vi "Autonomous_Execution.vi"(0 "Queue Key":refnum<queue>, 5 "Autonomous_Queue":refnum<queue>, 11 "error in":errorcluster) -> (6 "Done":bool)   [LabVIEW 2019]
uses:
  Queue_Key_Data.ctl
  Robot_Subsystems.ctl
  Subsystems/Drive/Drive_Cluster.ctl
  Subsystems/Drive/Drive_Control_States.ctl
  Subsystems/Drive/Drive_Orientation_States.ctl
  Subsystems/Intake/Intake_Cluster.ctl
  Subsystems/Intake/Intake_States.ctl
  Globals/Drive_Globals.vi
  Globals/Intake_Globals.vi
panel:
  in  "ignore previous (F)":bool
  in  "timeout in ms (-1)":i32=15
  out "notifiers out":refnum<notifier>[](array[refnum])
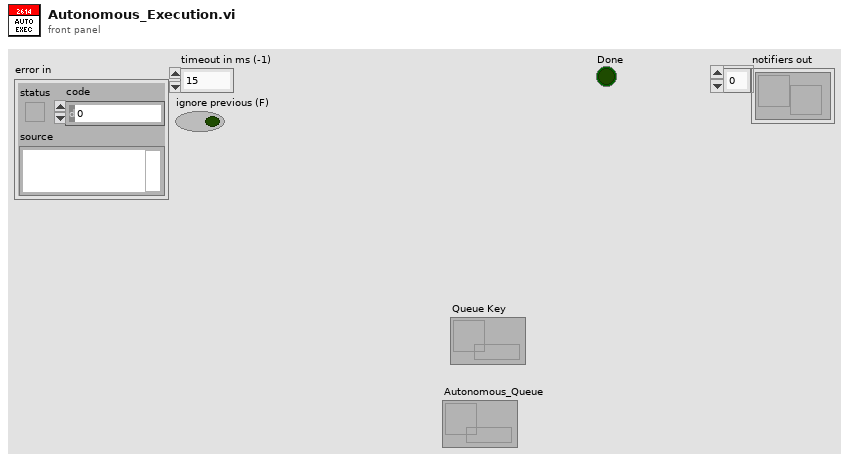
[diagram p1: front panel]
types:
  T1 = typedef "Queue_Key_Data.ctl" = cluster{"Operation Notifier":refnum<notifier>, "Subsystem":string, "Concurrent":bool}
  T2 = typedef "Robot_Subsystems.ctl" = cluster{"Drive_Cluster":T3, "Intake_Cluster":T6}
  T3 = typedef "Drive_Cluster.ctl" = cluster{"Control_State":T4, "Vertical_Throttle":dbl, "Lateral_Throttle":dbl, "Rotational_Throttle":dbl, "Strafe_In_Deadband":bool, "Rotation_In_Deadband":bool, "Orientation_State":T5, "Parameters":dbl[], "Step":i32, "Auto_Notifier":refnum<notifier>, "PathName":string}
  T4 = typedef "Drive_Control_States.ctl" = enum16{"No-Op", "Manual_Control", "Command_DriveDistanceAtAngle", "Command_DrivePath"}
  T5 = typedef "Drive_Orientation_States.ctl" = enum16{"Robot-Oriented", "Field-Oriented"}
  T6 = typedef "Intake_Cluster.ctl" = cluster{"Control_State":T7, "Intake_On":bool, "Intake_Extended":bool, "Intake_Throttle":dbl, "Auto_Notifier":refnum<notifier>, "Step":dbl, "Outtake":bool, "Parameters":dbl[]}
  T7 = typedef "Intake_States.ctl" = enum16{"Manual_Throttle", "Manual_Single_Speed", "Compliant_Intake", "Command_RunIntake"}
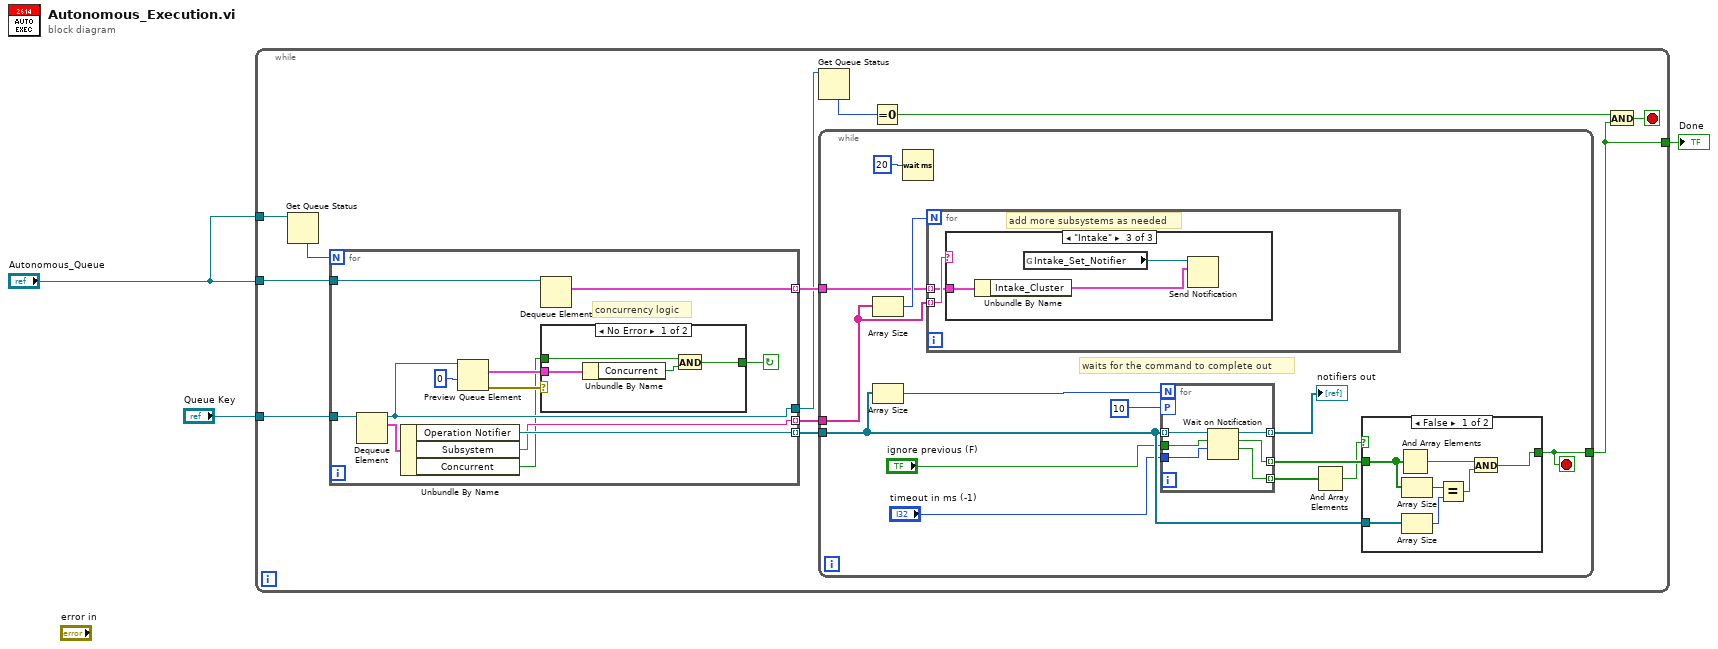
[diagram p0: block diagram]
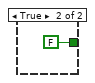
[diagram p2: hidden frame]
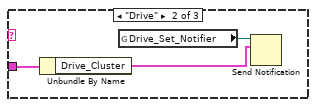
[diagram p4: hidden frame]
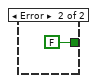
[diagram p5: hidden frame]
diagram:
  n1 = while {
    tunnel: "Queue Key" -> [w14]
    tunnel: "Autonomous_Queue" -> [w15]
    tunnel: "Autonomous_Queue" -> [w6]
    tunnel: [w4] -> w2
    stop <- w7 stop-if-true
    n2 = Get Queue Status(queue=w6) -> (# elements in queue=w9:i32)  [unwired: 2 in, 7 out]
    n3 = for {
      N: w9 -> [_]
      tunnel: w15 -> [w57]
      tunnel: w14 -> [w63]
      tunnel: [w54] -> w10 mode=indexing
      tunnel: [w58] -> w5
      tunnel: [w53] -> w12 mode=indexing
      tunnel: [w56] -> w11 mode=indexing
      stop <- w59 continue-if-true
      # "concurrency logic"
      n4 = Dequeue Element(queue=w63) -> (queue out=w58:refnum<queue>, element=w55:T1)  [unwired: 2 in, 2 out]
      n5 = Unbundle By Name(w55) -> ("Operation Notifier"=w54:refnum<notifier>, "Subsystem"=w53:string, "Concurrent"=w52:bool)
      n6 = Preview Queue Element(queue=w58, timeout in ms (-1)=0) -> (element=w62:T1, error out=w60:errorcluster)  [unwired: 1 in, 2 out]
      n7 = Dequeue Element(queue=w57) -> (element=w56:T2)  [unwired: 2 in, 3 out]
      n8 = case shown="No Error" w60 {
        tunnel: w62 -> [w65 _]
        tunnel: [w67 FALSE] -> w59
        tunnel: w52 -> [w66 _]
        frame No Error {
          n9 = Unbundle By Name(w65) -> ("Concurrent"=w64:bool)
          n10 = And(x=w66, y=w64) -> (x .and. y?=w67:bool)
        }
        frame Error {
        }
      }
    }
    n11 = Get Queue Status(queue=w5) -> (# elements in queue=w13:i32)  [unwired: 2 in, 7 out]
    n12 = while {
      tunnel: w12 -> [w24]
      tunnel: w11 -> [w23]
      tunnel: w10 -> [w25]
      tunnel: [w26] -> w4
      stop <- w26 stop-if-true
      # "waits for the command to complete out"
      n13 = Array Size(array=w24) -> (size(s)=w27:i32)
      n14 = Array Size(array=w25) -> (size(s)=w19:i32)
      n15 = Wait (ms)(milliseconds to wait=u32 20) -> ()  [unwired: 1 out]
      n16 = for {
        N: w27 -> [_]
        tunnel: w24 -> [w45] mode=indexing
        tunnel: w23 -> [w44] mode=indexing
        # "add more subsystems as needed"
        n17 = case shown="\"Intake\"" w45 {
          tunnel: w44 -> [_ w48 w51]
          frame "No_Op", Default {
          }
          frame "Drive" {
            n18 = Unbundle By Name(w48) -> ("Drive_Cluster"=w47:T3)
            n19 = global read "Drive_Globals.vi" "Drive_Set_Notifier"() -> (w46:refnum<notifier>)
            n20 = Send Notification(notification=w47, notifier=w46) -> ()  [unwired: 1 in, 2 out]
          }
          frame "Intake" {
            n21 = Unbundle By Name(w51) -> ("Intake_Cluster"=w50:T6)
            n22 = global read "Intake_Globals.vi" "Intake_Set_Notifier"() -> (w49:refnum<notifier>)
            n23 = Send Notification(notification=w50, notifier=w49) -> ()  [unwired: 1 in, 2 out]
          }
        }
      }
      n24 = for {
        N: w19 -> [_]
        tunnel: w25 -> [w35] mode=indexing
        workers-P: 10 -> [_]
        tunnel: "timeout in ms (-1)" -> [w34]
        tunnel: "ignore previous (F)" -> [w33]
        tunnel: [w32] -> w22 mode=indexing
        tunnel: [w31] -> w29 mode=indexing
        tunnel: [w30] -> w17 mode=indexing
        n25 = Wait on Notification(notifier=w35, ignore previous (F)=w33, timeout in ms (-1)=w34) -> (notifier out=w32:refnum<notifier>, notification=w31:bool, timed out?=w30:bool)  [unwired: 1 in, 1 out]
      }
      "notifiers out" <- w22
      n26 = And Array Elements(Boolean array=w17) -> (logical AND=w28:bool)
      n27 = case shown="False" w28 {
        tunnel: [w41 FALSE] -> w26
        tunnel: w29 -> [w40 _]
        tunnel: w25 -> [w39 _]
        frame False {
          n28 = And Array Elements(Boolean array=w40) -> (logical AND=w42:bool)
          n29 = Array Size(array=w40) -> (size(s)=w38:i32)
          n30 = Array Size(array=w39) -> (size(s)=w37:i32)
          n31 = Equal?(x=w38, y=w37) -> (x = y?=w36:bool)
          n32 = And(x=w42, y=w36) -> (x .and. y?=w41:bool)
        }
        frame True {
        }
      }
    }
    n33 = Equal To 0?(x=w13) -> (x = 0?=w8:bool)
    n34 = And(x=w8, y=w4) -> (x .and. y?=w7:bool)
  }
  "Done" <- w2
